vi "Drive Loop.vi"(1 "RobotDriveDevRef":T4={"DevStatus"={"status"=FALSE, "code"=0, "source"=""}, "Motors[]"=[], "Square Inputs"=FALSE, "Max Output"=1.0, "Isochronous"=FALSE}, 2 "Sonar":T1) -> ()   [LabVIEW 2012]
uses:
  <vilib>/Rock Robotics/WPI/RobotDrive/WPI_RobotDriveDevRef.ctl
  <vilib>/Rock Robotics/WPI/MotorControl/WPI_MotorControlDeviceRef.ctl
  <vilib>/Rock Robotics/SystemInterfaces/Typedef/FPGA_TypedefDigitalModule.ctl
  <vilib>/Rock Robotics/SystemInterfaces/DIO/FPGA_DIOPWMChannel.ctl
  <vilib>/Rock Robotics/WPI/PWM/WPI_PWMDeadband.ctl
  <vilib>/Rock Robotics/WPI/CAN/Jaguar/SubVIs/WPI_CANJaguar_ControlMode.ctl
  <vilib>/Rock Robotics/WPI/PWM/WPI_PWMTransform_ConPane.ctl
  <vilib>/Rock Robotics/WPI/AnalogChannel/WPI_AnalogChannelDevRef.ctl
  <vilib>/Rock Robotics/SystemInterfaces/Typedef/FPGA_TypedefAnalogModule.ctl
  <vilib>/Rock Robotics/SystemInterfaces/AI/FPGA_AIChannel.ctl
panel:
  in  "Drive Width":dbl=3.0
  in  "Drive Delay":dbl
  in  "Sonar Delay":dbl(knob)=0.22282942714120238 scale=0.0..1.0
  out "Detect":bool
  out "Sonar":dbl(graph)
  out "Dist":dbl
  in  "Thres Dist":dbl=26.0
  in  "Sonar Scale":dbl(knob)=102.7182978218157 scale=80.0..120.0
  in  "Sonar Offset":dbl(knob)=-0.020166607778801193 scale=-20.0..20.0
  in  "Auto Speed":dbl=0.52
  # "Pos values back up\nNeg values go forward"
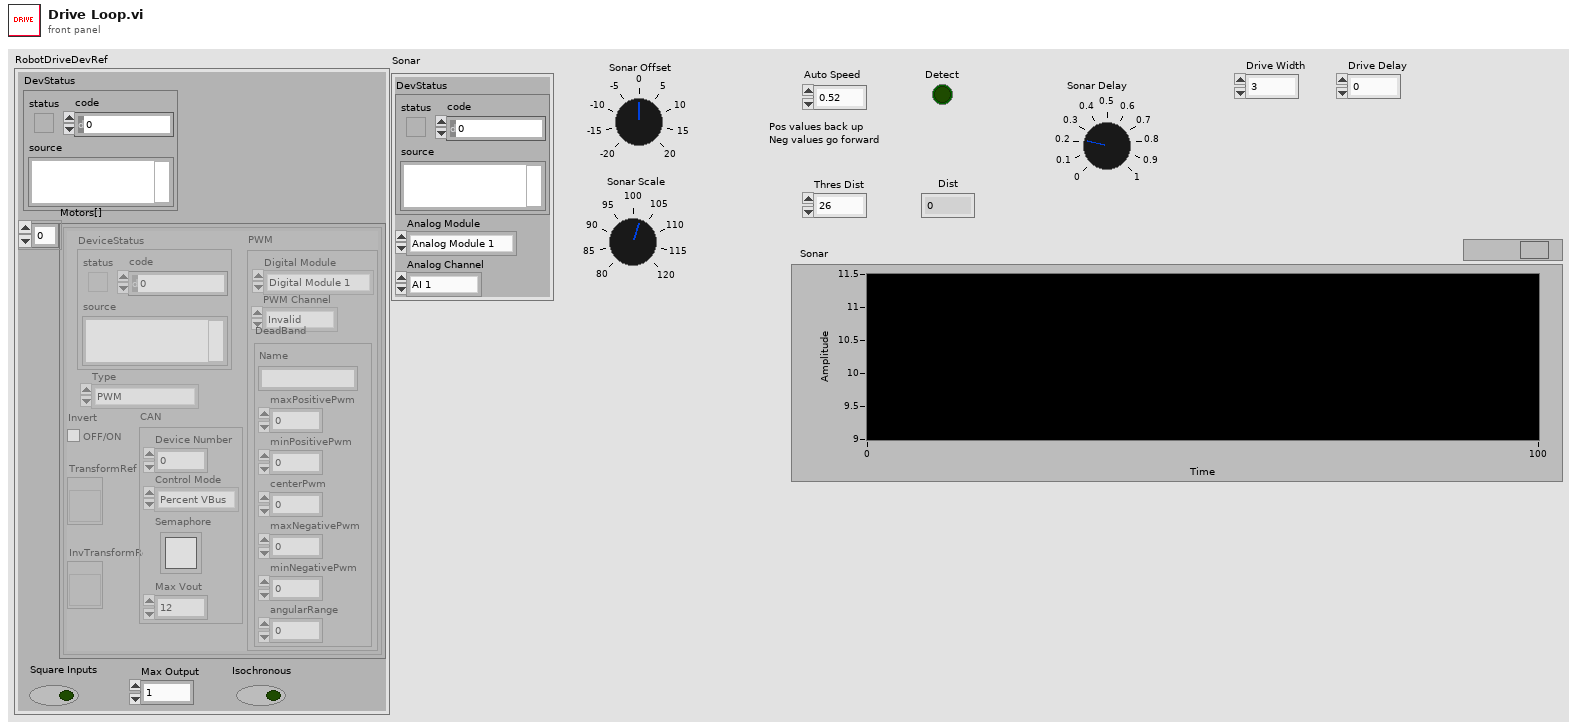
[diagram p1: front panel]
types:
  T1 = typedef "WPI_AnalogChannelDevRef.ctl" = cluster{"DevStatus":errorcluster, "Analog Module":T2, "Analog Channel":T3}
  T2 = typedef "FPGA_TypedefAnalogModule.ctl" = enum16{"Analog Module 1", "Analog Module 2"}
  T3 = typedef "FPGA_AIChannel.ctl" = enum8{"AI 1", "AI 2", "AI 3", "AI 4", "AI 5", "AI 6", "AI 7", "AI 8", "Invalid"}
  T4 = typedef "WPI_RobotDriveDevRef.ctl" = cluster{"DevStatus":errorcluster, "Motors[]":T5[], "Square Inputs":bool, "Max Output":dbl, "Isochronous":bool}
  T5 = typedef "WPI_MotorControlDeviceRef.ctl" = cluster{"DeviceStatus":errorcluster, "Type":enum16{"PWM", "CAN"}, "PWM":cluster{"Digital Module":T6, "PWM Channel":T7, "DeadBand":T8}, "CAN":cluster{"Device Number":u8, "Control Mode":T9, "Semaphore":T10, "Max Vout":dbl}, "Invert":bool, "TransformRef":T11, "InvTransformRef":T11}
  T6 = typedef "FPGA_TypedefDigitalModule.ctl" = enum16{"Digital Module 1", "Digital Module 2"}
  T7 = typedef "FPGA_DIOPWMChannel.ctl" = enum8{"PWM 1", "PWM 2", "PWM 3", "PWM 4", "PWM 5", "PWM 6", "PWM 7", "PWM 8", "PWM 9", "PWM 10", "Invalid"}
  T8 = typedef "WPI_PWMDeadband.ctl" = cluster{"Name":string, "maxPositivePwm":i32, "minPositivePwm":i32, "centerPwm":i32, "maxNegativePwm":i32, "minNegativePwm":i32, "angularRange":u16}
  T9 = typedef "WPI_CANJaguar_ControlMode.ctl" = enum8{"Percent VBus", "Current", "Speed", "Position", "Voltage"}
  T10 = typedef "Semaphore RefNum" = refnum<k1>
  T11 = typedef "WPI_PWMTransform_ConPane.ctl" = refnum<vi>
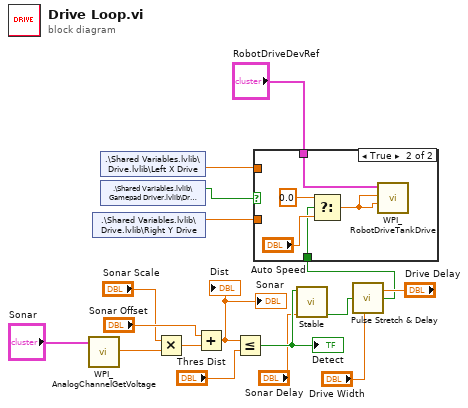
[diagram p0: block diagram]
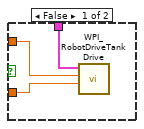
[diagram p2: hidden frame]
diagram:
  n1 = call <vilib>:"WPI_AnalogChannelGetVoltage.vi"("AIDeviceRef"="Sonar") -> ("Voltage"=w14:dbl)  [unwired: 1 in, 9 out]
  n2 = shared-variable ".\\Shared Variables.lvlib\\Drive.lvlib\\Right Y Drive"() -> (w3:dbl)  [unwired: 1 in, 1 out]
  n3 = shared-variable ".\\Shared Variables.lvlib\\Drive.lvlib\\Left X Drive"() -> (w4:dbl)  [unwired: 1 in, 1 out]
  n4 = shared-variable ".\\Shared Variables.lvlib\\Gamepad Driver.lvlib\\Dr Button 2"() -> (w5:bool)  [unwired: 1 in, 1 out]
  n5 = Multiply(x="Sonar Scale", y=w14) -> (x*y=w16:dbl)
  n6 = Add(x="Sonar Offset", y=w16) -> (x+y=w12:dbl)
  "Dist" <- w12
  "Sonar" <- w12
  n7 = Less Or Equal?(x=w12, y="Thres Dist") -> (x <= y?=w11:bool)
  "Detect" <- w11
  n8 = call "Stable.vi"("Eval Period (sec)"="Sonar Delay", "Signal Input"=w11) -> ("Stable"=w9:bool)  [unwired: 9 in]
  n9 = call "Pulse Stretch & Delay.vi"("Delay (sec)"="Drive Delay", "In"=w9, "Width (sec)"="Drive Width") -> ("Out"=w6:bool)  [unwired: 2 in]
  n10 = case shown="True" w5 {
    tunnel: "RobotDriveDevRef" -> [w20 w25]
    tunnel: w4 -> [w19 _]
    tunnel: w3 -> [w18 _]
    tunnel: w6 -> [_ w22]
    frame False {
      n11 = call <vilib>:"WPI_RobotDriveTankDrive.vi"("Right axis value"=w18, "Left axis value"=w19, "RobotDriveDevRef"=w20) -> ()  [unwired: 6 in, 3 out]
    }
    frame True {
      n12 = Select(t=0.0, s=w22, f="Auto Speed") -> (s? t:f=w21:dbl)
      n13 = call <vilib>:"WPI_RobotDriveTankDrive.vi"("Right axis value"=w21, "Left axis value"=w21, "RobotDriveDevRef"=w25) -> ()  [unwired: 6 in, 3 out]
    }
  }
